vi "nCr.vi"(1 "R":i32, 2 "N":i32) -> (0 "Combinations":i32)   [LabVIEW 2016]
uses:
  <vilib>/gmath/NI_Gmath.lvlib
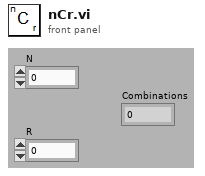
[diagram p1: front panel]
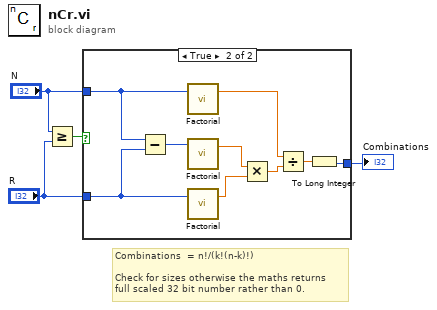
[diagram p0: block diagram]
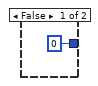
[diagram p2: hidden frame]
diagram:
  # "Combinations  = n!/(k!(n-k)!)\n\nCheck for sizes otherwise the maths returns\nfull scaled 32 bit number rather than 0."
  n1 = Greater Or Equal?(x="N", y="R") -> (x >= y?=w3:bool)
  n2 = case shown="True" w3 {
    tunnel: "N" -> [_ w14]
    tunnel: "R" -> [_ w13]
    tunnel: [0 w6] -> w4
    frame False {
    }
    frame True {
      n3 = Subtract(x=w14, y=w13) -> (x-y=w12:i32)
      n4 = call <vilib>:"Factorial.vi"("n"=w14) -> ("n!"=w8:dbl)  [unwired: 2 in]
      n5 = call <vilib>:"Factorial.vi"("n"=w12) -> ("n!"=w10:dbl)  [unwired: 2 in]
      n6 = call <vilib>:"Factorial.vi"("n"=w13) -> ("n!"=w11:dbl)  [unwired: 2 in]
      n7 = Multiply(x=w10, y=w11) -> (x*y=w9:dbl)
      n8 = Divide(x=w8, y=w9) -> (x/y=w7:dbl)
      n9 = To Long Integer(number=w7) -> (32bit integer=w6:i32)
    }
  }
  "Combinations" <- w4
